vi "3.1-Joystick Override.vi"() -> (0 "Numeric 2":fxp<+/-,19,4> format="%.17g", 1 "Numeric":fxp<+/-,19,4> format="%.17g", 2 "Joystick Setpoints":bool, 3 "Numeric 3":fxp<+/-,19,4> format="%.17g", 4 "Trig":bool)   [LabVIEW 2010]
uses:
  3.0-Global.vi
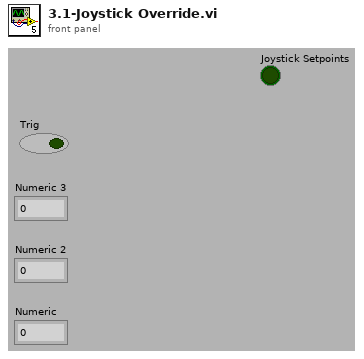
[diagram p1: front panel]
types:
  T1 = typedef "4.1.1-Act Joystick.ctl" = cluster{"Trig":bool, "2":bool, "3":bool, "4":bool, "5":bool, "6":bool, "7":bool, "8":bool, "9":bool, "10":bool, "11":bool, "Pitch":i32, "Ang":bool[], "Wheel":dbl, "Roll":i32, "Yaw":i32, "Left":i32, "Right":i32}
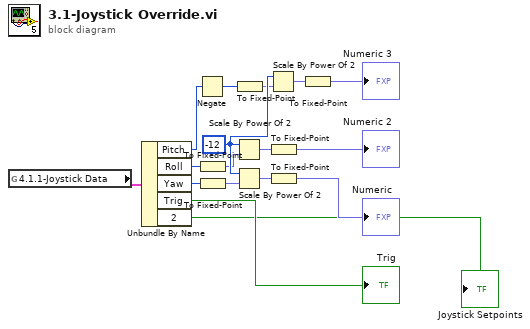
[diagram p0: block diagram]
diagram:
  w9 = -12 ("n")
  n1 = global read "3.0-Global.vi" "4.1.1-Joystick Data"() -> (w2:T1)
  n2 = Unbundle By Name(w2) -> ("Pitch"=w3:i32, "Roll"=w4:i32, "Yaw"=w5:i32, "Trig"=→"Trig":bool, "2"=→"Joystick Setpoints":bool)
  n3 = Negate(x=w3) -> (-x=w13:i32)
  n4 = To Fixed-Point(number=w4) -> (fixed-point=w7:fxp<+/-,32,16>)  [unwired: 1 in]
  n5 = To Fixed-Point(number=w5) -> (fixed-point=w8:fxp<+/-,32,16>)  [unwired: 1 in]
  n6 = Scale By Power Of 2(n=w9, x=w7) -> (x*2^n=w12:fxp<+/-,32,16>)
  n7 = Scale By Power Of 2(n=w9, x=w8) -> (x*2^n=w11:fxp<+/-,32,16>)
  n8 = To Fixed-Point(number=w13) -> (fixed-point=w6:fxp<+/-,32,16>)  [unwired: 1 in]
  n9 = Scale By Power Of 2(n=w9, x=w6) -> (x*2^n=w10:fxp<+/-,32,16>)
  n10 = To Fixed-Point(number=w12) -> (fixed-point=→"Numeric 2":fxp<+/-,19,4>)  [unwired: 1 in]
  n11 = To Fixed-Point(number=w11) -> (fixed-point=→"Numeric":fxp<+/-,19,4>)  [unwired: 1 in]
  n12 = To Fixed-Point(number=w10) -> (fixed-point=→"Numeric 3":fxp<+/-,19,4>)  [unwired: 1 in]
